vi "AD7747_Read.vi"(3 "error in":errorcluster, 4 "DUT Mask Array (All)":bool[][](array[boolean])=[[TRUE, TRUE, TRUE, TRUE, TRUE, TRUE, TRUE, TRUE, TRUE, TRUE, TRUE, TRUE, TRUE, TRUE, TRUE, TRUE, FALSE, FALSE, FALSE, FALSE, FALSE, FALSE, FALSE, FALSE, FALSE, FALSE, FALSE, FALSE, FALSE, FALSE, FALSE, FALSE], [TRUE, TRUE, TRUE, TRUE, TRUE, TRUE, TRUE, TRUE, TRUE, TRUE, TRUE, TRUE, TRUE, TRUE, TRUE, TRUE, FALSE, FALSE, FALSE, FALSE, FALSE, FALSE, FALSE, FALSE, FALSE, FALSE, FALSE, FALSE, FALSE, FALSE, FALSE, FALSE], [FALSE, FALSE, FALSE, FALSE, FALSE, FALSE, FALSE, FALSE, FALSE, FALSE, FALSE, FALSE, FALSE, FALSE, FALSE, FALSE, TRUE, FALSE, FALSE, FALSE, FALSE, FALSE, TRUE, FALSE, FALSE, FALSE, FALSE, FALSE, FALSE, FALSE, FALSE, TRUE], [FALSE, FALSE, FALSE, FALSE, FALSE, FALSE, FALSE, FALSE, FALSE, FALSE, FALSE, FALSE, FALSE, FALSE, FALSE, FALSE, TRUE, FALSE, FALSE, FALSE, FALSE, FALSE, TRUE, FALSE, FALSE, FALSE, FALSE, FALSE, FALSE, FALSE, FALSE, TRUE]], 5 "Log (T)":bool=TRUE) -> (0 "error Out":errorcluster, 2 "AD7747 Values":string[][](table))   [LabVIEW 2012]
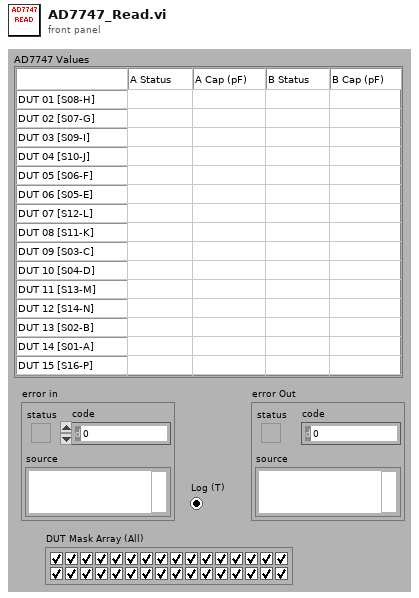
[diagram p1: front panel]
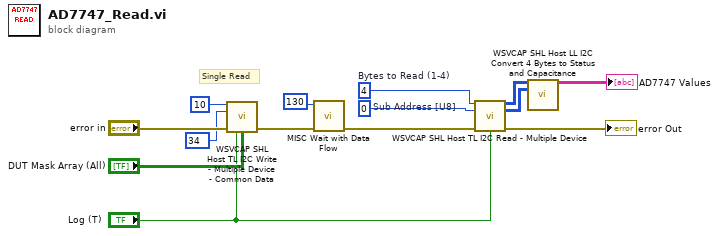
[diagram p0: block diagram]
diagram:
  w11 = u8 4  # Bytes to Read (1-4)
  w12 = u8 0  # Sub Address [U8]
  # "Single Read"
  n1 = call "WSVCAP SHL Host TL I2C Write - Multiple Device - Common Data.vi"("Sub Address"=u8 10, "Data Out [U8]"=u8 34 ("Sub Address"), "error in"="error in", "Log (T)"="Log (T)", "DUT Mask Array (All)"="DUT Mask Array (All)") -> ("error out"=w1:errorcluster)  [unwired: 10 in]
  n2 = call "MISC Wait with Data Flow.vi"("Error In (no error)"=w1, "Wait Time (500ms)"=u32 130 ("milliseconds to wait")) -> ("Error Out"=w3:errorcluster)  [unwired: 7 in, 2 out]
  n3 = call "WSVCAP SHL Host TL I2C Read - Multiple Device.vi"("Bytes to Read (1-4)"=w11, "Sub Address [U8]"=w12, "error in"=w3, "Log (T)"="Log (T)") -> ("A1-A16 Read Data [U8]"=w10:u8[][], "B1-B16 Read Data [U8]"=w9:u8[][], "error out"=→"error Out":errorcluster)  [unwired: 9 in]
  n4 = call "WSVCAP SHL Host LL I2C Convert 4 Bytes to Status and Capacitance.vi"("A1-A16 Read Data [U8]"=w10, "B1-B16 Read Data [U8]"=w9) -> ("AD7747 Values"=→"AD7747 Values":string[][])  [unwired: 13 in]
